vi "kormeedb_upload_api.vi"(0 "上传信息输入":T1, 1 "要上传的数据":string[](array[string]), 6 "数据存在则替换?":bool=TRUE) -> (5 "error in":errorcluster, 14 "操作结果":string, 19 "error out":errorcluster)   [LabVIEW 2015]
uses:
  global/tcp_conn.vi
panel:
  out "json数据（utf8）":string
  out "response":string
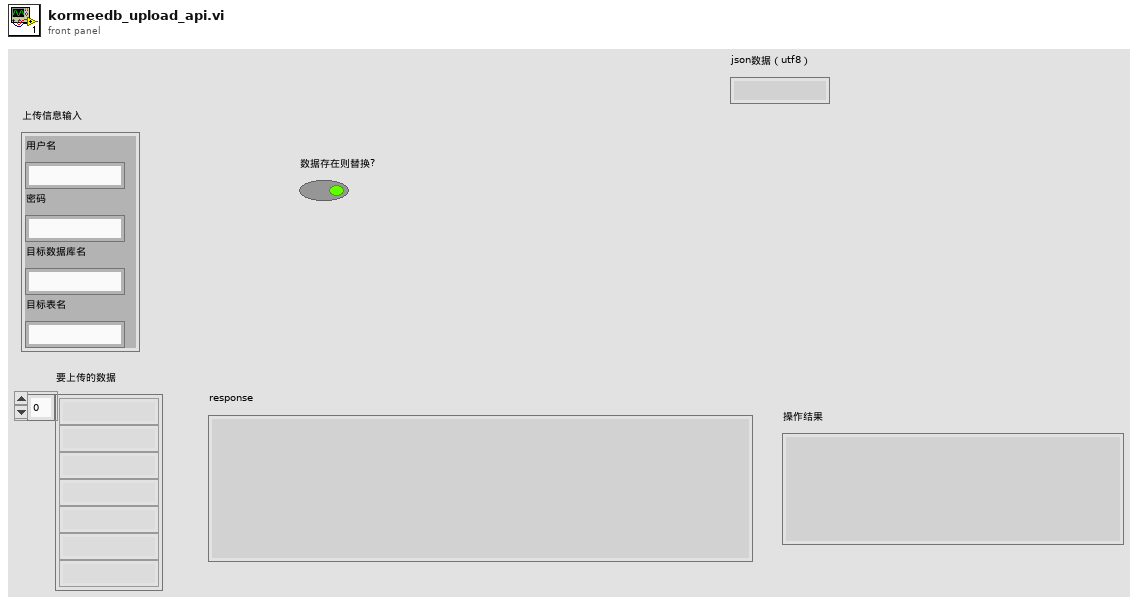
[diagram p1: front panel]
types:
  T1 = cluster{"用户名":string, "密码":string, "目标数据库名":string, "目标表名":string}
  T2 = enum16{"Standard", "Buffered", "CRLF", "Immediate"}
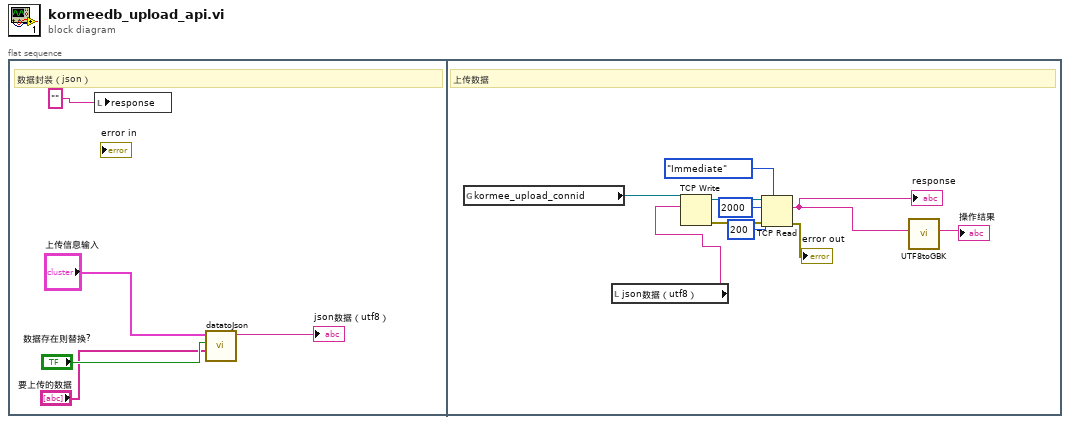
[diagram p0: block diagram]
diagram:
  n1 = flat-sequence {
    frame #0 {
      # "数据封装（json）"
      n2 = local write "response"("") -> ()
      n3 = call "datatoJson.vi"("要上传的数据"="要上传的数据", "数据存在则替换?"="数据存在则替换?", "上传信息输入"="上传信息输入") -> ("utf-8 text"=→"json数据（utf8）":string)  [unwired: 8 in]
    }
    frame #1 {
      # "上传数据"
      n4 = global read "tcp_conn.vi" "kormee_upload_connid"() -> (w15:refnum<k5>)
      n5 = local read "json数据（utf8）"() -> (w7:string)
      n6 = TCP Write(connection ID=w15, data in=w7) -> (connection ID out=w14:refnum<k5>, error out=w13:errorcluster)  [unwired: 2 in, 1 out]
      n7 = TCP Read(connection ID=w14, bytes to read=2000 ("读取的字节"), error in (no error)=w13, 7:T2."Immediate" ("模式（标准）"), 9:200 ("超时毫秒(25000)")) -> (data out=w9:string, error out=→"error out":errorcluster)  [unwired: 1 out]
      "response" <- w9
      n8 = call "UTF8toGBK.vi"("UTF-8"=w9) -> ("GBK"=→"操作结果":string)  [unwired: 10 in]
    }
  }
